vi "show_tag_status_2.vi"(11 "file path (dialog if empty)":path=path "C:/RFID/status.csv") -> (2 "train_passes_text":string, 3 "Output Cluster":T1)   [LabVIEW 2015]
uses:
  <vilib>/Utility/file.llb/Read Delimited Spreadsheet (string).vi
panel:
  out "all rows":string[][](array[string])
  in  "Cluster":T1
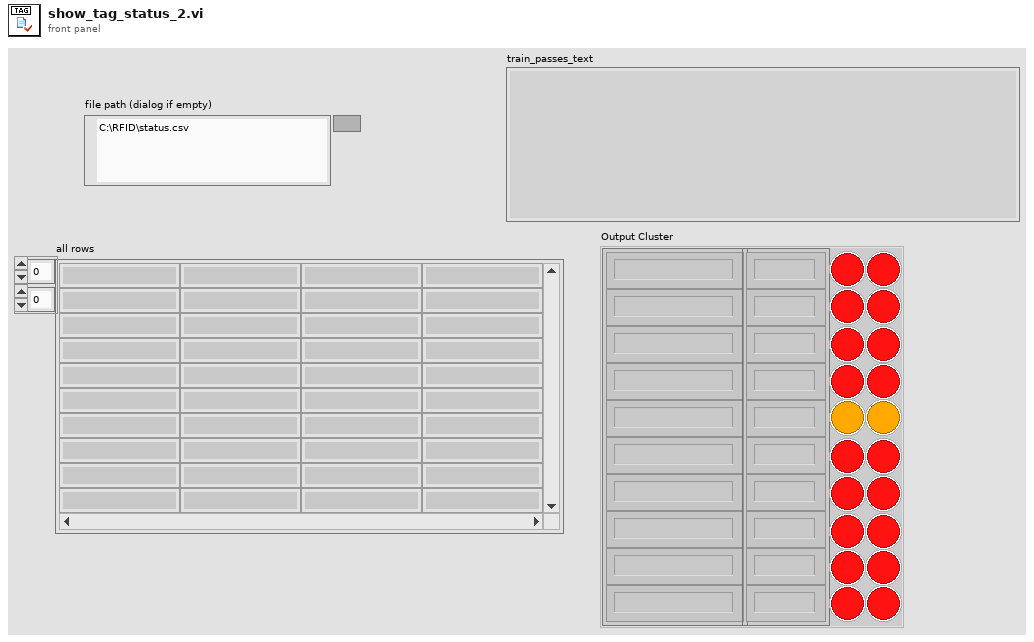
[diagram p1: front panel]
types:
  T1 = cluster{"Array 1":string[], "Array 2":string[], "Tag1":bool, "Tag2":bool, "Tag3":bool, "Tag4":bool, "Tag5":bool, "Tag6":bool, "Tag7":bool, "Tag 8":bool, "Tag9":bool, "Tag10":bool, "Tag101":bool, "Tag11":bool, "Tag21":bool, "Tag31":bool, "Tag41":bool, "Tag51":bool, "Tag61":bool, "Tag71":bool, "Tag81":bool, "Tag91":bool}
  T2 = enum16{"open", "replace", "create", "open or create", "replace or create", "replace or create with confirmation"}
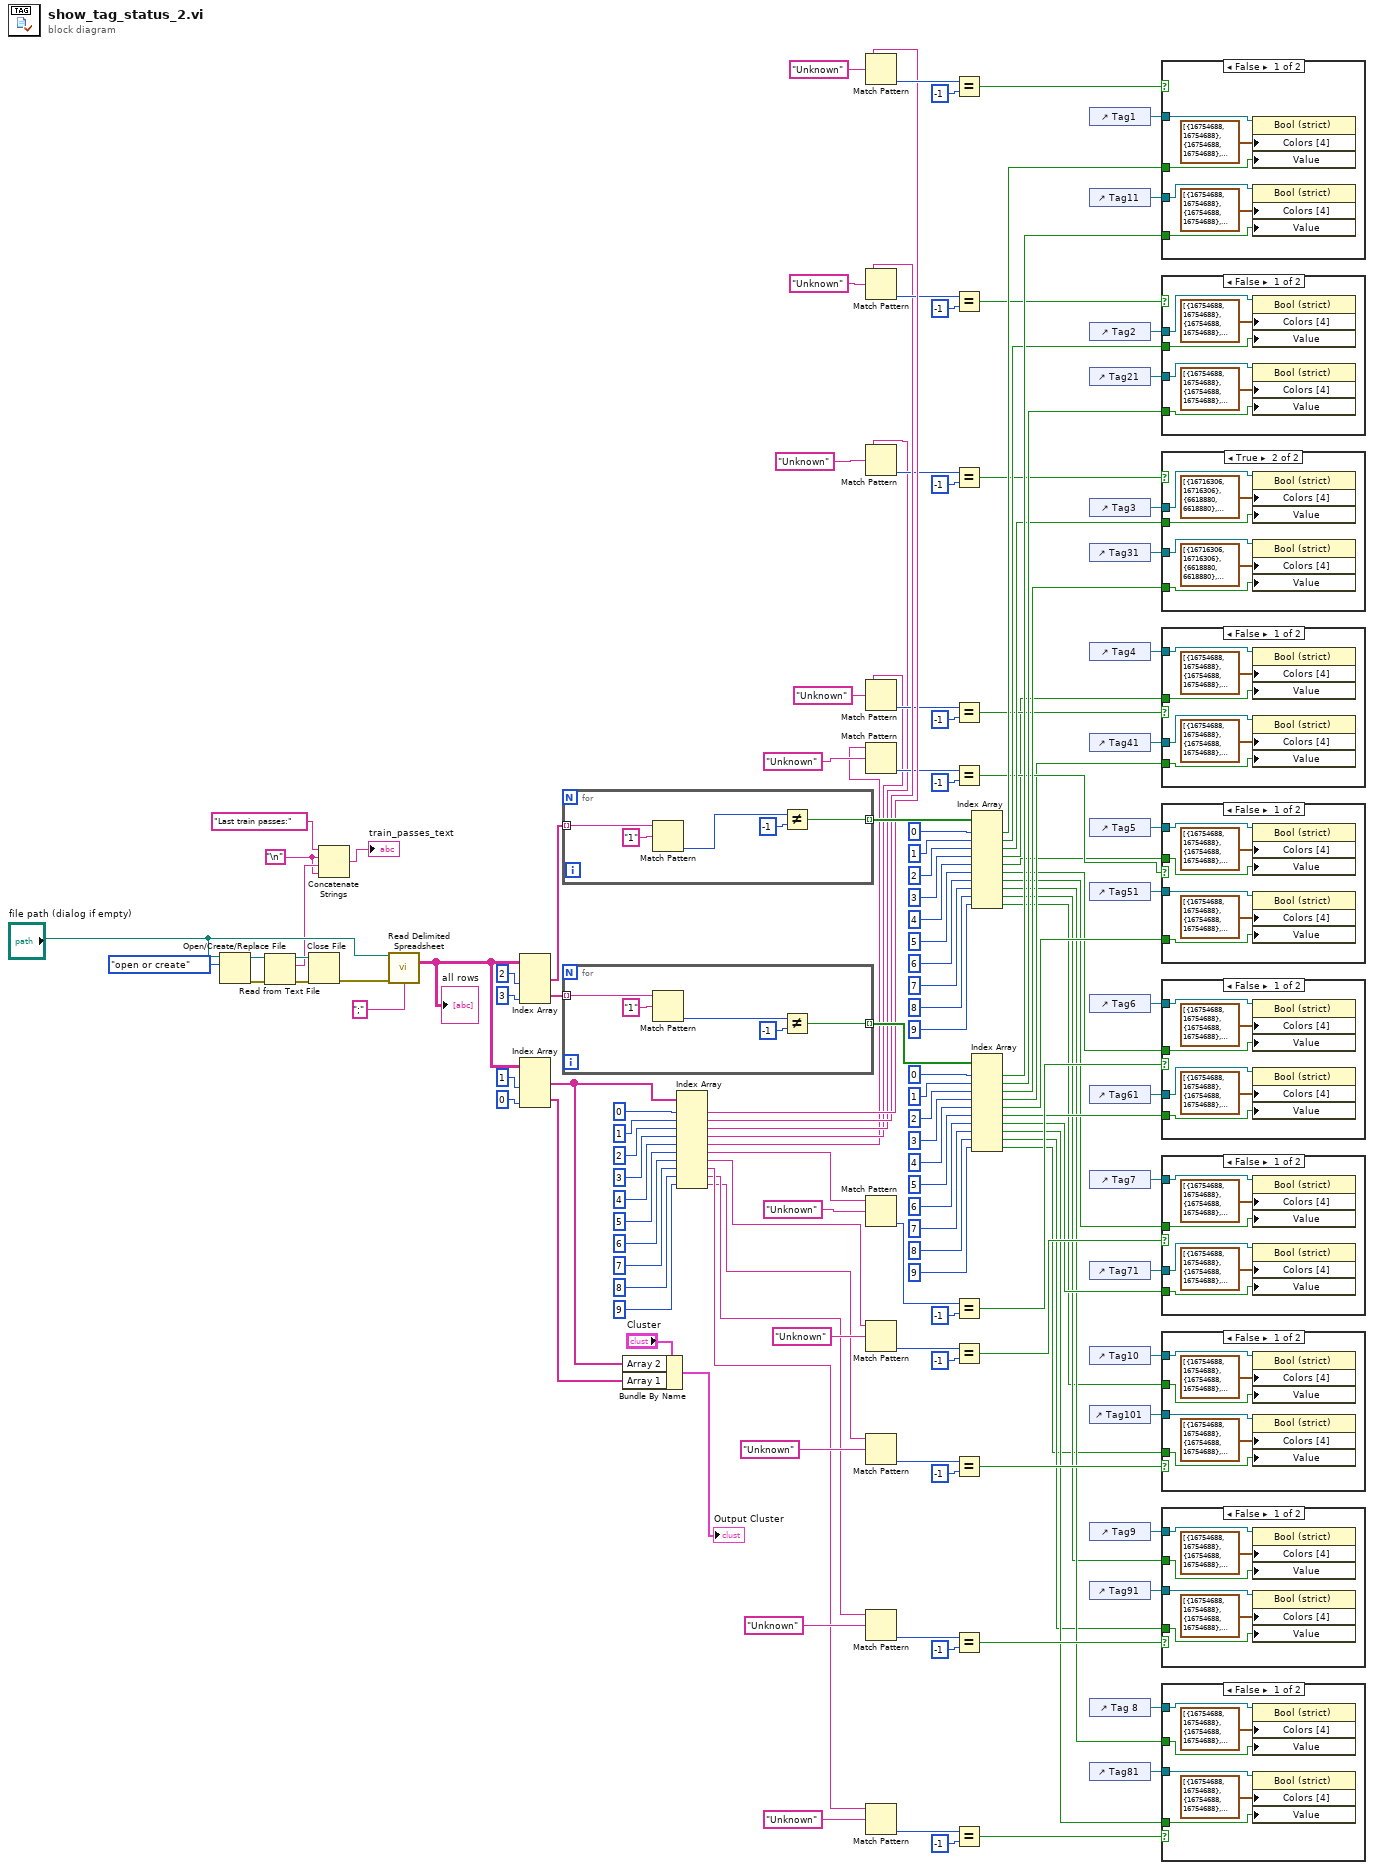
[diagram p0: block diagram]
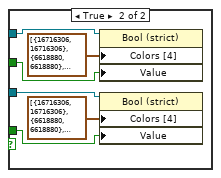
[diagram p2: hidden frame]
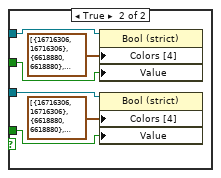
[diagram p3: hidden frame]
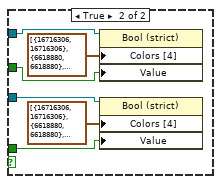
[diagram p4: hidden frame]
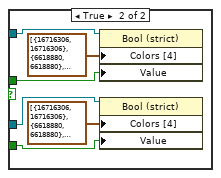
[diagram p5: hidden frame]
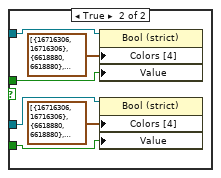
[diagram p6: hidden frame]
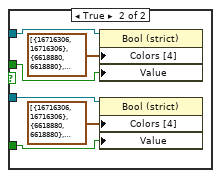
[diagram p7: hidden frame]
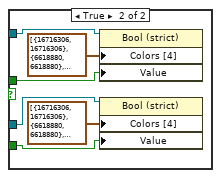
[diagram p8: hidden frame]
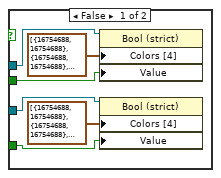
[diagram p9: hidden frame]
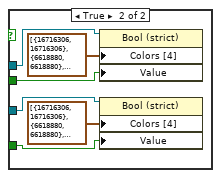
[diagram p10: hidden frame]
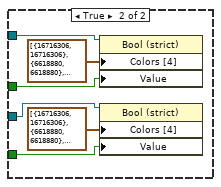
[diagram p11: hidden frame]
diagram:
  w1 = "\n"
  n1 = Open/Create/Replace File(file path (use dialog)="file path (dialog if empty)", operation (0:open)=T2."open or create") -> (refnum out=w6:refnum<file>, error out=w8:errorcluster)  [unwired: 4 in, 1 out]
  n2 = Read from Text File(file (use dialog)=w6, error in=w8) -> (refnum out=w5:refnum<file>, text=w4:string, error out=w7:errorcluster)  [unwired: 2 in, 1 out]
  n3 = Close File(refnum=w5, error in=w7) -> (error out=w11:errorcluster)  [unwired: 1 out]
  n4 = Concatenate Strings("Last train passes:", w1, w4, w1) -> (→"train_passes_text":string)
  n5 = call-poly <vilib>:"Read Delimited Spreadsheet.vi"("file path (dialog if empty)"="file path (dialog if empty)", "error in (no error)"=w11, "delimiter (\\t)"=";" ("delimiter (\\t)")) -> ("all rows"=w138:string[][])  [unwired: 7 in, 5 out]
  "all rows" <- w138
  n6 = Index Array(array=w138, index (col) #1=2 ("index (col)"), index (col) #2=3 ("index (row)")) -> (element #1=w137:string[], element #2=w140:string[])  [unwired: 2 in]
  n7 = Index Array(array=w138, index (col) #1=1 ("index"), index (col) #2=0 ("index (col)")) -> (element #1=w12:string[], element #2=w13:string[])  [unwired: 2 in]
  n8 = for {
    tunnel: w137 -> [w147] mode=indexing
    tunnel: [w146] -> w112 mode=indexing
    n9 = Match Pattern(string=w147, regular expression="1" ("element")) -> (offset past match=w148:i32)  [unwired: 1 in, 3 out]
    n10 = Not Equal?(x=w148, y=-1) -> (x != y?=w146:bool)
  }
  n11 = for {
    tunnel: w140 -> [w153] mode=indexing
    tunnel: [w151] -> w100 mode=indexing
    n12 = Match Pattern(string=w153, regular expression="1" ("element")) -> (offset past match=w152:i32)  [unwired: 1 in, 3 out]
    n13 = Not Equal?(x=w152, y=-1) -> (x != y?=w151:bool)
  }
  n14 = Bundle By Name(cluster="Cluster", "Array 2"=w12, "Array 1"=w13) -> (→"Output Cluster":T1)
  n15 = Index Array(array=w12, index #1=0 ("index"), index #2=1 ("index"), index #3=2 ("index"), index #4=3 ("index"), index #5=4 ("index"), index #6=5 ("index"), index #7=6 ("index"), index #8=7 ("index"), index #9=8 ("index"), index #10=9 ("index")) -> (element #1=w99:string, element #2=w91:string, element #3=w38:string, element #4=w37:string, element #5=w36:string, element #6=w35:string, element #7=w34:string, element #8=w33:string, element #9=w32:string, element #10=w31:string)
  n16 = Match Pattern(string=w99, regular expression="Unknown") -> (offset past match=w135:i32)  [unwired: 1 in, 3 out]
  n17 = Match Pattern(string=w91, regular expression="Unknown") -> (offset past match=w94:i32)  [unwired: 1 in, 3 out]
  n18 = Match Pattern(string=w38, regular expression="Unknown") -> (offset past match=w81:i32)  [unwired: 1 in, 3 out]
  n19 = Match Pattern(string=w37, regular expression="Unknown") -> (offset past match=w78:i32)  [unwired: 1 in, 3 out]
  n20 = Match Pattern(string=w36, regular expression="Unknown") -> (offset past match=w75:i32)  [unwired: 1 in, 3 out]
  n21 = Match Pattern(string=w35, regular expression="Unknown") -> (offset past match=w72:i32)  [unwired: 1 in, 3 out]
  n22 = Match Pattern(string=w34, regular expression="Unknown") -> (offset past match=w69:i32)  [unwired: 1 in, 3 out]
  n23 = Match Pattern(string=w31, regular expression="Unknown") -> (offset past match=w60:i32)  [unwired: 1 in, 3 out]
  n24 = Match Pattern(string=w32, regular expression="Unknown") -> (offset past match=w63:i32)  [unwired: 1 in, 3 out]
  n25 = Match Pattern(string=w33, regular expression="Unknown") -> (offset past match=w66:i32)  [unwired: 1 in, 3 out]
  n26 = Equal?(x=w135, y=-1) -> (x = y?=w133:bool)
  n27 = Equal?(x=w94, y=-1) -> (x = y?=w92:bool)
  n28 = Equal?(x=w81, y=-1) -> (x = y?=w14:bool)
  n29 = Equal?(x=w78, y=-1) -> (x = y?=w52:bool)
  n30 = Equal?(x=w75, y=-1) -> (x = y?=w53:bool)
  n31 = Equal?(x=w72, y=-1) -> (x = y?=w54:bool)
  n32 = Equal?(x=w69, y=-1) -> (x = y?=w55:bool)
  n33 = Equal?(x=w60, y=-1) -> (x = y?=w58:bool)
  n34 = Equal?(x=w63, y=-1) -> (x = y?=w57:bool)
  n35 = Equal?(x=w66, y=-1) -> (x = y?=w56:bool)
  n36 = Index Array(array=w112, index #1=0 ("index"), index #2=1 ("index"), index #3=2 ("index"), index #4=3 ("index"), index #5=4 ("index"), index #6=5 ("index"), index #7=6 ("index"), index #8=7 ("index"), index #9=8 ("index"), index #10=9 ("index")) -> (element #1=w98:bool, element #2=w90:bool, element #3=w83:bool, element #4=w30:bool, element #5=w28:bool, element #6=w26:bool, element #7=w24:bool, element #8=w22:bool, element #9=w20:bool, element #10=w16:bool)
  n37 = Index Array(array=w100, index #1=0 ("index"), index #2=1 ("index"), index #3=2 ("index"), index #4=3 ("index"), index #5=4 ("index"), index #6=5 ("index"), index #7=6 ("index"), index #8=7 ("index"), index #9=8 ("index"), index #10=9 ("index")) -> (element #1=w96:bool, element #2=w89:bool, element #3=w84:bool, element #4=w29:bool, element #5=w27:bool, element #6=w25:bool, element #7=w23:bool, element #8=w21:bool, element #9=w17:bool, element #10=w15:bool)
  n38 = control-ref of="Tag1"() -> (w132:refnum<vi>)
  n39 = control-ref of="Tag11"() -> (w97:refnum<vi>)
  n40 = control-ref of="Tag2"() -> (w88:refnum<vi>)
  n41 = control-ref of="Tag21"() -> (w87:refnum<vi>)
  n42 = control-ref of="Tag3"() -> (w86:refnum<vi>)
  n43 = control-ref of="Tag31"() -> (w85:refnum<vi>)
  n44 = control-ref of="Tag4"() -> (w51:refnum<vi>)
  n45 = control-ref of="Tag41"() -> (w50:refnum<vi>)
  n46 = control-ref of="Tag5"() -> (w48:refnum<vi>)
  n47 = control-ref of="Tag51"() -> (w49:refnum<vi>)
  n48 = control-ref of="Tag6"() -> (w47:refnum<vi>)
  n49 = control-ref of="Tag61"() -> (w46:refnum<vi>)
  n50 = control-ref of="Tag7"() -> (w45:refnum<vi>)
  n51 = control-ref of="Tag71"() -> (w44:refnum<vi>)
  n52 = control-ref of="Tag10"() -> (w39:refnum<vi>)
  n53 = control-ref of="Tag101"() -> (w40:refnum<vi>)
  n54 = control-ref of="Tag9"() -> (w19:refnum<vi>)
  n55 = control-ref of="Tag91"() -> (w18:refnum<vi>)
  n56 = control-ref of="Tag 8"() -> (w43:refnum<vi>)
  n57 = control-ref of="Tag81"() -> (w42:refnum<vi>)
  n58 = case shown="False" w133 {
    tunnel: w132 -> [w159 w167]
    tunnel: w98 -> [w160 w165]
    tunnel: w97 -> [w156 w163]
    tunnel: w96 -> [w157 w162]
    frame False {
      n59 = property class="Bool (strict)"(reference=w159, "Colors [4]"=cluster{"Color Box":u32, "Color Box 2":u32}[] [{"Color Box"=16754688, "Color Box 2"=16754688}, {"Color Box"=16754688, "Color Box 2"=16754688}, {"Color Box"=1985280, "Color Box 2"=1985280}, {"Color Box"=6618880, "Color Box 2"=6618880}] ("Array 2"), "Value"=w160) -> ()  [unwired: 1 in, 2 out]
      n60 = property class="Bool (strict)"(reference=w156, "Colors [4]"=cluster{"Color Box":u32, "Color Box 2":u32}[] [{"Color Box"=16754688, "Color Box 2"=16754688}, {"Color Box"=16754688, "Color Box 2"=16754688}, {"Color Box"=1985280, "Color Box 2"=1985280}, {"Color Box"=6618880, "Color Box 2"=6618880}] ("Array 2"), "Value"=w157) -> ()  [unwired: 1 in, 2 out]
    }
    frame True {
      n61 = property class="Bool (strict)"(reference=w167, "Colors [4]"=cluster{"Color Box":u32, "Color Box 2":u32}[] [{"Color Box"=16716306, "Color Box 2"=16716306}, {"Color Box"=6618880, "Color Box 2"=6618880}, {"Color Box"=1985280, "Color Box 2"=1985280}, {"Color Box"=6618880, "Color Box 2"=6618880}] ("Array 2"), "Value"=w165) -> ()  [unwired: 1 in, 2 out]
      n62 = property class="Bool (strict)"(reference=w163, "Colors [4]"=cluster{"Color Box":u32, "Color Box 2":u32}[] [{"Color Box"=16716306, "Color Box 2"=16716306}, {"Color Box"=6618880, "Color Box 2"=6618880}, {"Color Box"=1985280, "Color Box 2"=1985280}, {"Color Box"=6618880, "Color Box 2"=6618880}] ("Array 2"), "Value"=w162) -> ()  [unwired: 1 in, 2 out]
    }
  }
  n63 = case shown="False" w92 {
    tunnel: w88 -> [w171 w179]
    tunnel: w90 -> [w172 w177]
    tunnel: w87 -> [w168 w175]
    tunnel: w89 -> [w169 w174]
    frame False {
      n64 = property class="Bool (strict)"(reference=w171, "Colors [4]"=cluster{"Color Box":u32, "Color Box 2":u32}[] [{"Color Box"=16754688, "Color Box 2"=16754688}, {"Color Box"=16754688, "Color Box 2"=16754688}, {"Color Box"=1985280, "Color Box 2"=1985280}, {"Color Box"=6618880, "Color Box 2"=6618880}] ("Array 2"), "Value"=w172) -> ()  [unwired: 1 in, 2 out]
      n65 = property class="Bool (strict)"(reference=w168, "Colors [4]"=cluster{"Color Box":u32, "Color Box 2":u32}[] [{"Color Box"=16754688, "Color Box 2"=16754688}, {"Color Box"=16754688, "Color Box 2"=16754688}, {"Color Box"=1985280, "Color Box 2"=1985280}, {"Color Box"=6618880, "Color Box 2"=6618880}] ("Array 2"), "Value"=w169) -> ()  [unwired: 1 in, 2 out]
    }
    frame True {
      n66 = property class="Bool (strict)"(reference=w179, "Colors [4]"=cluster{"Color Box":u32, "Color Box 2":u32}[] [{"Color Box"=16716306, "Color Box 2"=16716306}, {"Color Box"=6618880, "Color Box 2"=6618880}, {"Color Box"=1985280, "Color Box 2"=1985280}, {"Color Box"=6618880, "Color Box 2"=6618880}] ("Array 2"), "Value"=w177) -> ()  [unwired: 1 in, 2 out]
      n67 = property class="Bool (strict)"(reference=w175, "Colors [4]"=cluster{"Color Box":u32, "Color Box 2":u32}[] [{"Color Box"=16716306, "Color Box 2"=16716306}, {"Color Box"=6618880, "Color Box 2"=6618880}, {"Color Box"=1985280, "Color Box 2"=1985280}, {"Color Box"=6618880, "Color Box 2"=6618880}] ("Array 2"), "Value"=w174) -> ()  [unwired: 1 in, 2 out]
    }
  }
  n68 = case shown="True" w14 {
    tunnel: w86 -> [w183 w191]
    tunnel: w83 -> [w184 w189]
    tunnel: w85 -> [w180 w187]
    tunnel: w84 -> [w181 w186]
    frame False {
      n69 = property class="Bool (strict)"(reference=w183, "Colors [4]"=cluster{"Color Box":u32, "Color Box 2":u32}[] [{"Color Box"=16754688, "Color Box 2"=16754688}, {"Color Box"=16754688, "Color Box 2"=16754688}, {"Color Box"=1985280, "Color Box 2"=1985280}, {"Color Box"=6618880, "Color Box 2"=6618880}] ("Array 2"), "Value"=w184) -> ()  [unwired: 1 in, 2 out]
      n70 = property class="Bool (strict)"(reference=w180, "Colors [4]"=cluster{"Color Box":u32, "Color Box 2":u32}[] [{"Color Box"=16754688, "Color Box 2"=16754688}, {"Color Box"=16754688, "Color Box 2"=16754688}, {"Color Box"=1985280, "Color Box 2"=1985280}, {"Color Box"=6618880, "Color Box 2"=6618880}] ("Array 2"), "Value"=w181) -> ()  [unwired: 1 in, 2 out]
    }
    frame True {
      n71 = property class="Bool (strict)"(reference=w191, "Colors [4]"=cluster{"Color Box":u32, "Color Box 2":u32}[] [{"Color Box"=16716306, "Color Box 2"=16716306}, {"Color Box"=6618880, "Color Box 2"=6618880}, {"Color Box"=1985280, "Color Box 2"=1985280}, {"Color Box"=6618880, "Color Box 2"=6618880}] ("Array 2"), "Value"=w189) -> ()  [unwired: 1 in, 2 out]
      n72 = property class="Bool (strict)"(reference=w187, "Colors [4]"=cluster{"Color Box":u32, "Color Box 2":u32}[] [{"Color Box"=16716306, "Color Box 2"=16716306}, {"Color Box"=6618880, "Color Box 2"=6618880}, {"Color Box"=1985280, "Color Box 2"=1985280}, {"Color Box"=6618880, "Color Box 2"=6618880}] ("Array 2"), "Value"=w186) -> ()  [unwired: 1 in, 2 out]
    }
  }
  n73 = case shown="False" w52 {
    tunnel: w51 -> [w195 w203]
    tunnel: w30 -> [w196 w201]
    tunnel: w50 -> [w192 w199]
    tunnel: w29 -> [w193 w198]
    frame False {
      n74 = property class="Bool (strict)"(reference=w195, "Colors [4]"=cluster{"Color Box":u32, "Color Box 2":u32}[] [{"Color Box"=16754688, "Color Box 2"=16754688}, {"Color Box"=16754688, "Color Box 2"=16754688}, {"Color Box"=1985280, "Color Box 2"=1985280}, {"Color Box"=6618880, "Color Box 2"=6618880}] ("Array 2"), "Value"=w196) -> ()  [unwired: 1 in, 2 out]
      n75 = property class="Bool (strict)"(reference=w192, "Colors [4]"=cluster{"Color Box":u32, "Color Box 2":u32}[] [{"Color Box"=16754688, "Color Box 2"=16754688}, {"Color Box"=16754688, "Color Box 2"=16754688}, {"Color Box"=1985280, "Color Box 2"=1985280}, {"Color Box"=6618880, "Color Box 2"=6618880}] ("Array 2"), "Value"=w193) -> ()  [unwired: 1 in, 2 out]
    }
    frame True {
      n76 = property class="Bool (strict)"(reference=w203, "Colors [4]"=cluster{"Color Box":u32, "Color Box 2":u32}[] [{"Color Box"=16716306, "Color Box 2"=16716306}, {"Color Box"=6618880, "Color Box 2"=6618880}, {"Color Box"=1985280, "Color Box 2"=1985280}, {"Color Box"=6618880, "Color Box 2"=6618880}] ("Array 2"), "Value"=w201) -> ()  [unwired: 1 in, 2 out]
      n77 = property class="Bool (strict)"(reference=w199, "Colors [4]"=cluster{"Color Box":u32, "Color Box 2":u32}[] [{"Color Box"=16716306, "Color Box 2"=16716306}, {"Color Box"=6618880, "Color Box 2"=6618880}, {"Color Box"=1985280, "Color Box 2"=1985280}, {"Color Box"=6618880, "Color Box 2"=6618880}] ("Array 2"), "Value"=w198) -> ()  [unwired: 1 in, 2 out]
    }
  }
  n78 = case shown="False" w53 {
    tunnel: w48 -> [w207 w215]
    tunnel: w28 -> [w208 w213]
    tunnel: w49 -> [w204 w211]
    tunnel: w27 -> [w205 w210]
    frame False {
      n79 = property class="Bool (strict)"(reference=w207, "Colors [4]"=cluster{"Color Box":u32, "Color Box 2":u32}[] [{"Color Box"=16754688, "Color Box 2"=16754688}, {"Color Box"=16754688, "Color Box 2"=16754688}, {"Color Box"=1985280, "Color Box 2"=1985280}, {"Color Box"=6618880, "Color Box 2"=6618880}] ("Array 2"), "Value"=w208) -> ()  [unwired: 1 in, 2 out]
      n80 = property class="Bool (strict)"(reference=w204, "Colors [4]"=cluster{"Color Box":u32, "Color Box 2":u32}[] [{"Color Box"=16754688, "Color Box 2"=16754688}, {"Color Box"=16754688, "Color Box 2"=16754688}, {"Color Box"=1985280, "Color Box 2"=1985280}, {"Color Box"=6618880, "Color Box 2"=6618880}] ("Array 2"), "Value"=w205) -> ()  [unwired: 1 in, 2 out]
    }
    frame True {
      n81 = property class="Bool (strict)"(reference=w215, "Colors [4]"=cluster{"Color Box":u32, "Color Box 2":u32}[] [{"Color Box"=16716306, "Color Box 2"=16716306}, {"Color Box"=6618880, "Color Box 2"=6618880}, {"Color Box"=1985280, "Color Box 2"=1985280}, {"Color Box"=6618880, "Color Box 2"=6618880}] ("Array 2"), "Value"=w213) -> ()  [unwired: 1 in, 2 out]
      n82 = property class="Bool (strict)"(reference=w211, "Colors [4]"=cluster{"Color Box":u32, "Color Box 2":u32}[] [{"Color Box"=16716306, "Color Box 2"=16716306}, {"Color Box"=6618880, "Color Box 2"=6618880}, {"Color Box"=1985280, "Color Box 2"=1985280}, {"Color Box"=6618880, "Color Box 2"=6618880}] ("Array 2"), "Value"=w210) -> ()  [unwired: 1 in, 2 out]
    }
  }
  n83 = case shown="False" w54 {
    tunnel: w47 -> [w219 w227]
    tunnel: w26 -> [w220 w225]
    tunnel: w46 -> [w216 w223]
    tunnel: w25 -> [w217 w222]
    frame False {
      n84 = property class="Bool (strict)"(reference=w219, "Colors [4]"=cluster{"Color Box":u32, "Color Box 2":u32}[] [{"Color Box"=16754688, "Color Box 2"=16754688}, {"Color Box"=16754688, "Color Box 2"=16754688}, {"Color Box"=1985280, "Color Box 2"=1985280}, {"Color Box"=6618880, "Color Box 2"=6618880}] ("Array 2"), "Value"=w220) -> ()  [unwired: 1 in, 2 out]
      n85 = property class="Bool (strict)"(reference=w216, "Colors [4]"=cluster{"Color Box":u32, "Color Box 2":u32}[] [{"Color Box"=16754688, "Color Box 2"=16754688}, {"Color Box"=16754688, "Color Box 2"=16754688}, {"Color Box"=1985280, "Color Box 2"=1985280}, {"Color Box"=6618880, "Color Box 2"=6618880}] ("Array 2"), "Value"=w217) -> ()  [unwired: 1 in, 2 out]
    }
    frame True {
      n86 = property class="Bool (strict)"(reference=w227, "Colors [4]"=cluster{"Color Box":u32, "Color Box 2":u32}[] [{"Color Box"=16716306, "Color Box 2"=16716306}, {"Color Box"=6618880, "Color Box 2"=6618880}, {"Color Box"=1985280, "Color Box 2"=1985280}, {"Color Box"=6618880, "Color Box 2"=6618880}] ("Array 2"), "Value"=w225) -> ()  [unwired: 1 in, 2 out]
      n87 = property class="Bool (strict)"(reference=w223, "Colors [4]"=cluster{"Color Box":u32, "Color Box 2":u32}[] [{"Color Box"=16716306, "Color Box 2"=16716306}, {"Color Box"=6618880, "Color Box 2"=6618880}, {"Color Box"=1985280, "Color Box 2"=1985280}, {"Color Box"=6618880, "Color Box 2"=6618880}] ("Array 2"), "Value"=w222) -> ()  [unwired: 1 in, 2 out]
    }
  }
  n88 = case shown="False" w55 {
    tunnel: w45 -> [w231 w239]
    tunnel: w24 -> [w232 w237]
    tunnel: w44 -> [w228 w235]
    tunnel: w23 -> [w229 w234]
    frame False {
      n89 = property class="Bool (strict)"(reference=w231, "Colors [4]"=cluster{"Color Box":u32, "Color Box 2":u32}[] [{"Color Box"=16754688, "Color Box 2"=16754688}, {"Color Box"=16754688, "Color Box 2"=16754688}, {"Color Box"=1985280, "Color Box 2"=1985280}, {"Color Box"=6618880, "Color Box 2"=6618880}] ("Array 2"), "Value"=w232) -> ()  [unwired: 1 in, 2 out]
      n90 = property class="Bool (strict)"(reference=w228, "Colors [4]"=cluster{"Color Box":u32, "Color Box 2":u32}[] [{"Color Box"=16754688, "Color Box 2"=16754688}, {"Color Box"=16754688, "Color Box 2"=16754688}, {"Color Box"=1985280, "Color Box 2"=1985280}, {"Color Box"=6618880, "Color Box 2"=6618880}] ("Array 2"), "Value"=w229) -> ()  [unwired: 1 in, 2 out]
    }
    frame True {
      n91 = property class="Bool (strict)"(reference=w239, "Colors [4]"=cluster{"Color Box":u32, "Color Box 2":u32}[] [{"Color Box"=16716306, "Color Box 2"=16716306}, {"Color Box"=6618880, "Color Box 2"=6618880}, {"Color Box"=1985280, "Color Box 2"=1985280}, {"Color Box"=6618880, "Color Box 2"=6618880}] ("Array 2"), "Value"=w237) -> ()  [unwired: 1 in, 2 out]
      n92 = property class="Bool (strict)"(reference=w235, "Colors [4]"=cluster{"Color Box":u32, "Color Box 2":u32}[] [{"Color Box"=16716306, "Color Box 2"=16716306}, {"Color Box"=6618880, "Color Box 2"=6618880}, {"Color Box"=1985280, "Color Box 2"=1985280}, {"Color Box"=6618880, "Color Box 2"=6618880}] ("Array 2"), "Value"=w234) -> ()  [unwired: 1 in, 2 out]
    }
  }
  n93 = case shown="False" w58 {
    tunnel: w39 -> [w243 w251]
    tunnel: w16 -> [w244 w249]
    tunnel: w40 -> [w240 w247]
    tunnel: w15 -> [w241 w246]
    frame False {
      n94 = property class="Bool (strict)"(reference=w243, "Colors [4]"=cluster{"Color Box":u32, "Color Box 2":u32}[] [{"Color Box"=16754688, "Color Box 2"=16754688}, {"Color Box"=16754688, "Color Box 2"=16754688}, {"Color Box"=1985280, "Color Box 2"=1985280}, {"Color Box"=6618880, "Color Box 2"=6618880}] ("Array 2"), "Value"=w244) -> ()  [unwired: 1 in, 2 out]
      n95 = property class="Bool (strict)"(reference=w240, "Colors [4]"=cluster{"Color Box":u32, "Color Box 2":u32}[] [{"Color Box"=16754688, "Color Box 2"=16754688}, {"Color Box"=16754688, "Color Box 2"=16754688}, {"Color Box"=1985280, "Color Box 2"=1985280}, {"Color Box"=6618880, "Color Box 2"=6618880}] ("Array 2"), "Value"=w241) -> ()  [unwired: 1 in, 2 out]
    }
    frame True {
      n96 = property class="Bool (strict)"(reference=w251, "Colors [4]"=cluster{"Color Box":u32, "Color Box 2":u32}[] [{"Color Box"=16716306, "Color Box 2"=16716306}, {"Color Box"=6618880, "Color Box 2"=6618880}, {"Color Box"=1985280, "Color Box 2"=1985280}, {"Color Box"=6618880, "Color Box 2"=6618880}] ("Array 2"), "Value"=w249) -> ()  [unwired: 1 in, 2 out]
      n97 = property class="Bool (strict)"(reference=w247, "Colors [4]"=cluster{"Color Box":u32, "Color Box 2":u32}[] [{"Color Box"=16716306, "Color Box 2"=16716306}, {"Color Box"=6618880, "Color Box 2"=6618880}, {"Color Box"=1985280, "Color Box 2"=1985280}, {"Color Box"=6618880, "Color Box 2"=6618880}] ("Array 2"), "Value"=w246) -> ()  [unwired: 1 in, 2 out]
    }
  }
  n98 = case shown="False" w57 {
    tunnel: w19 -> [w255 w263]
    tunnel: w20 -> [w256 w261]
    tunnel: w18 -> [w252 w259]
    tunnel: w17 -> [w253 w258]
    frame False {
      n99 = property class="Bool (strict)"(reference=w255, "Colors [4]"=cluster{"Color Box":u32, "Color Box 2":u32}[] [{"Color Box"=16754688, "Color Box 2"=16754688}, {"Color Box"=16754688, "Color Box 2"=16754688}, {"Color Box"=1985280, "Color Box 2"=1985280}, {"Color Box"=6618880, "Color Box 2"=6618880}] ("Array 2"), "Value"=w256) -> ()  [unwired: 1 in, 2 out]
      n100 = property class="Bool (strict)"(reference=w252, "Colors [4]"=cluster{"Color Box":u32, "Color Box 2":u32}[] [{"Color Box"=16754688, "Color Box 2"=16754688}, {"Color Box"=16754688, "Color Box 2"=16754688}, {"Color Box"=1985280, "Color Box 2"=1985280}, {"Color Box"=6618880, "Color Box 2"=6618880}] ("Array 2"), "Value"=w253) -> ()  [unwired: 1 in, 2 out]
    }
    frame True {
      n101 = property class="Bool (strict)"(reference=w263, "Colors [4]"=cluster{"Color Box":u32, "Color Box 2":u32}[] [{"Color Box"=16716306, "Color Box 2"=16716306}, {"Color Box"=6618880, "Color Box 2"=6618880}, {"Color Box"=1985280, "Color Box 2"=1985280}, {"Color Box"=6618880, "Color Box 2"=6618880}] ("Array 2"), "Value"=w261) -> ()  [unwired: 1 in, 2 out]
      n102 = property class="Bool (strict)"(reference=w259, "Colors [4]"=cluster{"Color Box":u32, "Color Box 2":u32}[] [{"Color Box"=16716306, "Color Box 2"=16716306}, {"Color Box"=6618880, "Color Box 2"=6618880}, {"Color Box"=1985280, "Color Box 2"=1985280}, {"Color Box"=6618880, "Color Box 2"=6618880}] ("Array 2"), "Value"=w258) -> ()  [unwired: 1 in, 2 out]
    }
  }
  n103 = case shown="False" w56 {
    tunnel: w43 -> [w267 w275]
    tunnel: w22 -> [w268 w273]
    tunnel: w42 -> [w264 w271]
    tunnel: w21 -> [w265 w270]
    frame False {
      n104 = property class="Bool (strict)"(reference=w267, "Colors [4]"=cluster{"Color Box":u32, "Color Box 2":u32}[] [{"Color Box"=16754688, "Color Box 2"=16754688}, {"Color Box"=16754688, "Color Box 2"=16754688}, {"Color Box"=1985280, "Color Box 2"=1985280}, {"Color Box"=6618880, "Color Box 2"=6618880}] ("Array 2"), "Value"=w268) -> ()  [unwired: 1 in, 2 out]
      n105 = property class="Bool (strict)"(reference=w264, "Colors [4]"=cluster{"Color Box":u32, "Color Box 2":u32}[] [{"Color Box"=16754688, "Color Box 2"=16754688}, {"Color Box"=16754688, "Color Box 2"=16754688}, {"Color Box"=1985280, "Color Box 2"=1985280}, {"Color Box"=6618880, "Color Box 2"=6618880}] ("Array 2"), "Value"=w265) -> ()  [unwired: 1 in, 2 out]
    }
    frame True {
      n106 = property class="Bool (strict)"(reference=w275, "Colors [4]"=cluster{"Color Box":u32, "Color Box 2":u32}[] [{"Color Box"=16716306, "Color Box 2"=16716306}, {"Color Box"=6618880, "Color Box 2"=6618880}, {"Color Box"=1985280, "Color Box 2"=1985280}, {"Color Box"=6618880, "Color Box 2"=6618880}] ("Array 2"), "Value"=w273) -> ()  [unwired: 1 in, 2 out]
      n107 = property class="Bool (strict)"(reference=w271, "Colors [4]"=cluster{"Color Box":u32, "Color Box 2":u32}[] [{"Color Box"=16716306, "Color Box 2"=16716306}, {"Color Box"=6618880, "Color Box 2"=6618880}, {"Color Box"=1985280, "Color Box 2"=1985280}, {"Color Box"=6618880, "Color Box 2"=6618880}] ("Array 2"), "Value"=w270) -> ()  [unwired: 1 in, 2 out]
    }
  }
